vi "Print Dialog Test.vi"   [LabVIEW 2015, in "Win32 Util.lvlib"]
uses:
  LabSDL2/Source/Libraries/Win32 Util/Win32 Util.lvlib
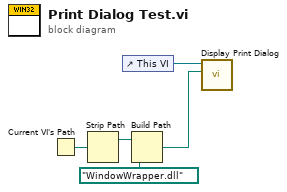
[diagram p0: block diagram]
diagram:
  n1 = Current VI's Path() -> (path=w4:path)
  n2 = Strip Path(path=w4) -> (stripped path=w3:path)  [unwired: 1 out]
  n3 = control-ref of="This VI"() -> (w5:refnum<vi>)
  n4 = Build Path(base path=w3, name or relative path=path "WindowWrapper.dll" ("WindowWrapper DLL Directory")) -> (appended path=w1:path)
  n5 = call "Display Print Dialog.vi"("WindowWrapper DLL Directory"=w1, "Main VI"=w5) -> ()  [unwired: 7 in, 3 out]
